vi "ClientSrv Server Access_srv.vi"(0 "method":T2=enum."test access", 1 "access level":T1, 5 "digest":string, 7 "certificate in":string, 11 "client version":string, 12 "access reason":string) -> (4 "server toolkit path":path, 8 "certificate/name out":string, 15 "error out":errorcluster)   [LabVIEW 2012]
doc: "This is a wrapper that makes a subset of the VI server access state object methods available for remote calling and also provides some client-only and composite methods. Certificate checks are performed on unsafe methods. The security scheme is outlined in the documentation of the security configuration user interface window."
uses:
  typedefs/t_ClientSrv Server Access Methods.ctl
  typedefs/t_ClientSrv Access Levels.ctl
  typedefs/t_ClientSrv Server Access State Methods.ctl
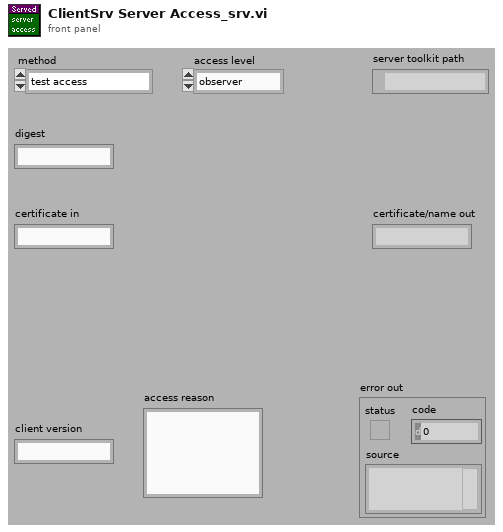
[diagram p1: front panel]
types:
  T1 = typedef "t_ClientSrv Access Levels.ctl" = enum16{"observer", "operator", "local"}
  T2 = typedef "t_ClientSrv Server Access Methods.ctl" = enum16{"validate access", "test access", "release access", "get name"}
  T3 = typedef "t_ClientSrv Server Access State Methods.ctl" = enum16{"initialize", "validate access", "test access", "release access", "get name", "dummy", "cleanup"}
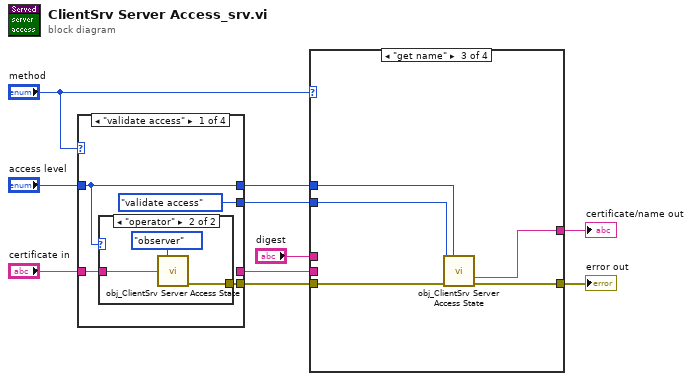
[diagram p0: block diagram]
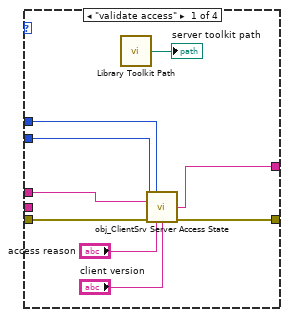
[diagram p2: hidden frame]
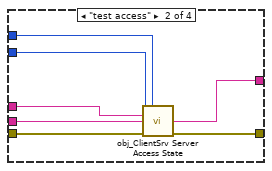
[diagram p3: hidden frame]
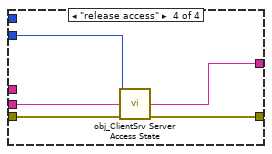
[diagram p4: hidden frame]
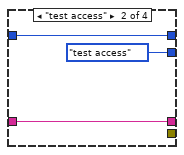
[diagram p6: hidden frame]
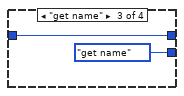
[diagram p7: hidden frame]
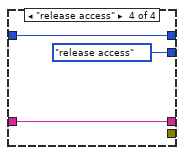
[diagram p8: hidden frame]
diagram:
  n1 = case shown="\"validate access\"" "method" {
    tunnel: [t_ClientSrv_Server_Access_State_Methods."validate access" ("method") t_ClientSrv_Server_Access_State_Methods."test access" ("method") t_ClientSrv_Server_Access_State_Methods."get name" ("method") t_ClientSrv_Server_Access_State_Methods."release access" ("method")] -> w4
    tunnel: "certificate in" -> [w13 w19 _ w24]
    tunnel: [_ w19 _ w24] -> w8
    tunnel: [w12 _ _ _] -> w5
    tunnel: "access level" -> [w11 w18 w21 w23]
    tunnel: [w11 w18 w21 w23] -> w1
    frame "validate access" {
      n2 = case shown="\"operator\"" w11 {
        tunnel: w13 -> [_ w16]
        tunnel: [_ w15] -> w12
        frame "observer", "local" {
        }
        frame "operator" {
          n3 = call "obj_ClientSrv Server Access State.vi"("access level"=t_ClientSrv_Access_Levels."observer", "certificate in"=w16) -> ("error out"=w15:errorcluster)  [unwired: 11 in, 2 out]
        }
      }
    }
    frame "test access" {
    }
    frame "get name" {
    }
    frame "release access" {
    }
  }
  n4 = case shown="\"get name\"" "method" {
    tunnel: [w27 w41 w46 w51] -> w10
    tunnel: w8 -> [_ w40 _ w50]
    tunnel: [w31 w39 w42 w49] -> w7
    tunnel: "digest" -> [w34 w38 _ _]
    tunnel: w5 -> [w33 w37 w45 w48]
    tunnel: w4 -> [w32 w36 w44 w47]
    tunnel: w1 -> [w29 w35 w43 _]
    frame "validate access" {
      n5 = call "Library Toolkit Path.vi"() -> ("absolute toolkit path"=→"server toolkit path":path)  [unwired: 15 in]
      n6 = call "obj_ClientSrv Server Access State.vi"("method (test access)"=w32, "access level"=w29, "digest"=w34, "error in (no error)"=w33, "access reason"="access reason", "client version"="client version") -> ("certificate out"=w31:string, "error out"=w27:errorcluster)  [unwired: 7 in, 1 out]
    }
    frame "test access" {
      n7 = call "obj_ClientSrv Server Access State.vi"("method (test access)"=w36, "access level"=w35, "digest"=w38, "certificate in"=w40, "error in (no error)"=w37) -> ("certificate out"=w39:string, "error out"=w41:errorcluster)  [unwired: 8 in, 1 out]
    }
    frame "get name" {
      n8 = call "obj_ClientSrv Server Access State.vi"("method (test access)"=w44, "access level"=w43, "error in (no error)"=w45) -> ("server name {get name}"=w42:string, "error out"=w46:errorcluster)  [unwired: 10 in, 1 out]
    }
    frame "release access" {
      n9 = call "obj_ClientSrv Server Access State.vi"("method (test access)"=w47, "certificate in"=w50, "error in (no error)"=w48) -> ("certificate out"=w49:string, "error out"=w51:errorcluster)  [unwired: 10 in, 1 out]
    }
  }
  "error out" <- w10
  "certificate/name out" <- w7
